vi "Initialize.vi"(8 "error in (no error)":errorcluster, 9 "Reset (True)":bool=TRUE, 10 "ID Query (True)":bool=TRUE, 11 "VISA resource name":refnum<visa-resource-name>) -> (0 "error out":errorcluster, 2 "Instrument Name":string, 3 "VISA resource name out":refnum<visa-resource-name>)   [LabVIEW 2020, in "Agilent 34405.lvlib"]
doc: "Establishes communication with the instrument and optionally performs an instrument identification query and/or an instrument reset. It also places the instrument in a default state needed for other instrument driver operations. Therefore, call this VI before calling other instrument driver VIs for this instrument. Generally, you need to call the Initialize VI only once at the beginning of an application."
uses:
  <instrlib>/Agilent 34405/Agilent 34405.lvlib
  <instrlib>/Agilent 34405/Private/Extended User Data.ctl
  <vilib>/regexp/Match Regular Expression.xnode
panel:
  # "(c) 2009 - 2015 National Instruments Corporation.  ALL RIGHTS RESERVED."
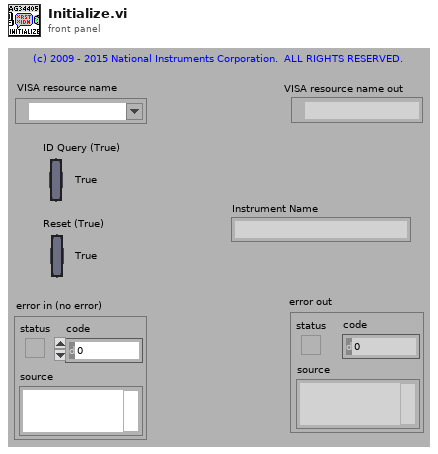
[diagram p1: front panel]
types:
  T1 = typedef "Agilent 34405.lvlib/Extended User Data.ctl" = cluster{"344XX Mode":u16, "Measurement Type":u16}
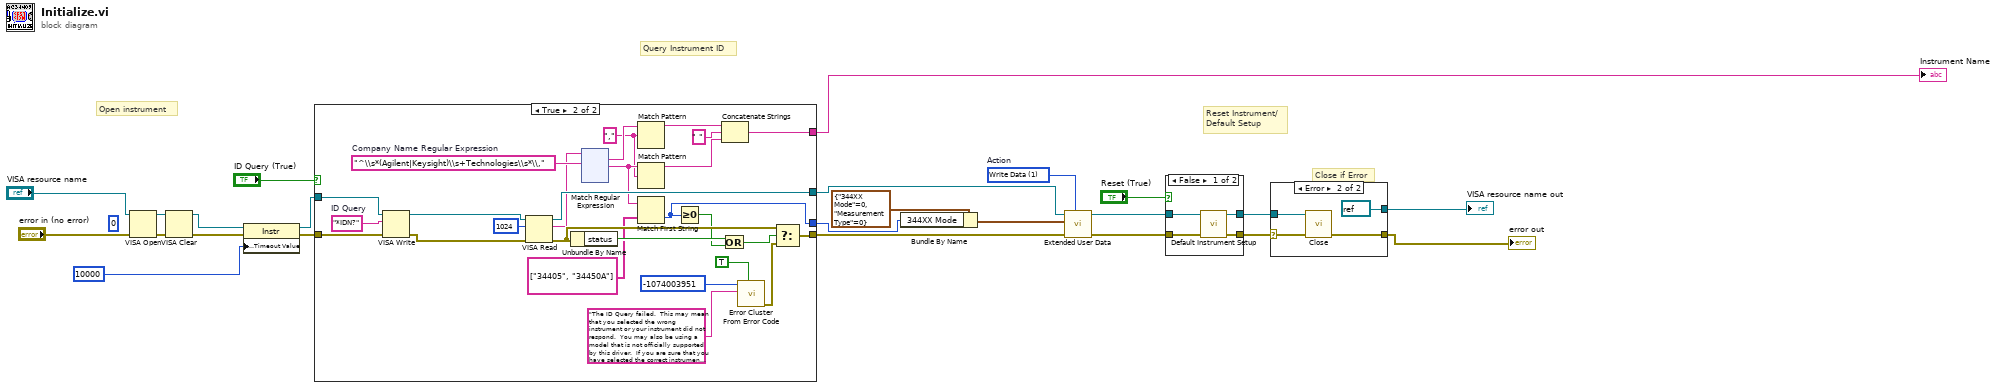
[diagram p0: block diagram]
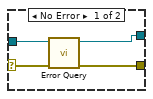
[diagram p2: hidden frame]
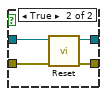
[diagram p3: hidden frame]
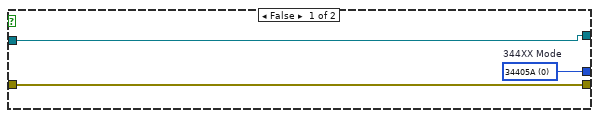
[diagram p4: hidden frame]
diagram:
  w5 = 1 items=["Read Data", "Write Data", "Clear Data", "Clear ALL Data"]  # Action
  (unwired) u32 0 ("access mode")
  # "Close if Error"
  # "Query Instrument ID"
  # "Reset Instrument/\nDefault Setup"
  # "Open instrument"
  n1 = VISA Open(error in (no error)="error in (no error)", VISA resource name="VISA resource name") -> (VISA resource name=w20:refnum<visa-resource-name>, error out=w19:errorcluster)  [unwired: 1 in, 2 out]
  n2 = VISA Clear(VISA resource name=w20, error in (no error)=w19) -> (VISA resource name out=w18:refnum<visa-resource-name>, error out=w17:errorcluster)
  n3 = property on="Property Node" class="Instr"(reference=w18, error in=w17, "General Settings:Timeout Value"=u32 10000) -> (reference out=w14:refnum<visa-resource-name>, error out=w13:errorcluster)
  n4 = case shown="True" "ID Query (True)" {
    tunnel: [w26 w54] -> w10
    tunnel: [w27 w51] -> w12
    tunnel: w14 -> [w27 w52]
    tunnel: w13 -> [w26 w53]
    tunnel: [w25 w37] -> w7
    tunnel: [_ w28] -> w4
    frame False {
      w25 = u16 0 items=["34405A", "34450A"]  # 344XX Mode
    }
    frame True {
      w32 = ","
      w36 = "^\\s*(Agilent|Keysight)\\s+Technologies\\s*\\,"  # Company Name Regular Expression
      w47 = "*IDN?"  # ID Query
      n5 = VISA Write(VISA resource name=w52, write buffer=w47, error in (no error)=w53) -> (VISA resource name out=w50:refnum<visa-resource-name>, error out=w49:errorcluster)  [unwired: 1 out]
      n6 = VISA Read(VISA resource name=w50, byte count=u32 1024, error in (no error)=w49) -> (VISA resource name out=w51:refnum<visa-resource-name>, read buffer=w35:string, error out=w42:errorcluster)  [unwired: 1 out]
      n7 = Unbundle By Name(w42) -> ("status"=w41:bool)
      n8 = xnode ("Match Regular Expression")("input string"=w35, "regular expression"=w36) -> ("whole match"=w33:string, "after match"=w34:string)  [unwired: 4 in, 3 out]
      n9 = Match Pattern(string=w33, regular expression=w32) -> (before substring=w31:string)  [unwired: 1 in, 3 out]
      n10 = Match Pattern(string=w34, regular expression=w32) -> (before substring=w30:string)  [unwired: 1 in, 3 out]
      n11 = Match First String(2:string[] ["34405", "34450A"] ("string array"), 3:w34) -> (0:w37:i32)  [unwired: 1 out]
      n12 = Greater Or Equal To 0?(x=w37) -> (x >= 0?=w40:bool)
      n13 = Or(x=w41, y=w40) -> (x .or. y?=w39:bool)
      n14 = Concatenate Strings(w31, " ", w30) -> (w28:string)
      n15 = call <vilib>:"Error Cluster From Error Code.vi"("show call chain? (False)"=TRUE, "error message (\"\")"="The ID Query failed.  This may mean that you selected the wrong instrument or your instrument did not respond.  You may also be using a model that is not officially supported by this driver.  If you are sure that you have selected the correct instrument and it is responding, try disabling the ID Query." ("Source (VI Name)"), "error code (0)"=-1074003951 ("Code")) -> ("error out"=w46:errorcluster)  [unwired: 1 in, 5 out]
      n16 = Select(t=w42, s=w39, f=w46) -> (s? t:f=w54:errorcluster)
    }
  }
  "Instrument Name" <- w4
  n17 = Bundle By Name(cluster=T1 {"344XX Mode"=0, "Measurement Type"=0} ("User Data In"), "344XX Mode"=w7) -> (w6:T1)
  n18 = call <instrlib>:"Extended User Data.vi"("Action"=w5, "error in (no error)"=w10, "User Data In"=w6, "VISA resource name in"=w12) -> ("error out"=w9:errorcluster, "VISA resource name out"=w11:refnum<visa-resource-name>)  [unwired: 6 out]
  n19 = case shown="False" "Reset (True)" {
    tunnel: w9 -> [w171 w173]
    tunnel: [w170 w176] -> w15
    tunnel: w11 -> [w172 w174]
    tunnel: [w169 w175] -> w16
    frame False {
      n20 = call <instrlib>:"Default Instrument Setup.vi"("error in (no error)"=w171, "VISA resource name"=w172) -> ("error out"=w170:errorcluster, "VISA resource name out"=w169:refnum<visa-resource-name>)  [unwired: 8 out]
    }
    frame True {
      n21 = call <instrlib>:"Reset.vi"("error in (no error)"=w173, "VISA resource name"=w174) -> ("error out"=w176:errorcluster, "VISA resource name out"=w175:refnum<visa-resource-name>)  [unwired: 8 out]
    }
  }
  n22 = case shown="Error" w15 {
    selector: w15 -> [w178 w182]
    tunnel: w16 -> [w177 w183]
    tunnel: [w180 refnum<visa-resource-name> refnum ("VISA resource name out")] -> w2
    tunnel: [w179 w184] -> w1
    frame No Error {
      n23 = call <instrlib>:"Error Query.vi"("error in (no error)"=w178, "VISA resource name"=w177) -> ("error out"=w179:errorcluster, "VISA resource name out"=w180:refnum<visa-resource-name>)  [unwired: 8 out]
    }
    frame Error {
      n24 = call <instrlib>:"Close.vi"("error in (no error)"=w182, "VISA resource name"=w183) -> ("error out"=w184:errorcluster)  [unwired: 9 out]
    }
  }
  "VISA resource name out" <- w2
  "error out" <- w1
